vi "target_exists.vi"(8 "error in":errorcluster, 10 "Target Name":string, 11 "vsd reference":refnum<k24>) -> (0 "error out":errorcluster, 1 "target if exists":refnum<k24>, 2 "Target Exists":bool, 3 "vsd reference out":refnum<k24>)   [LabVIEW 2020]
uses:
  NationalInstruments.VeriStand.SystemDefinitionAPI
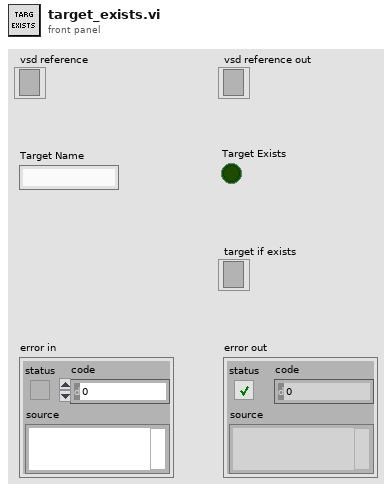
[diagram p1: front panel]
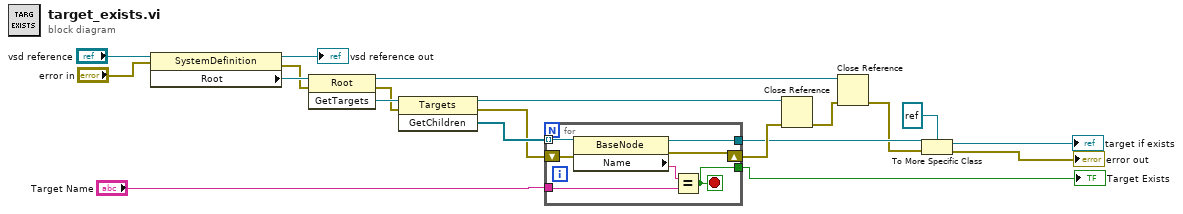
[diagram p0: block diagram]
diagram:
  n1 = property class="SystemDefinition"(reference="vsd reference", error in="error in") -> (reference out=→"vsd reference out":refnum<k24>, error out=w18:errorcluster, "Root"=w20:refnum<k24>)
  n2 = invoke class="Root" method="GetTargets"(reference=w20, error in=w18) -> (reference out=w12:refnum<k24>, error out=w6:errorcluster, "GetTargets"=w15:refnum<k24>)  [unwired: 1 in]
  n3 = invoke class="Targets" method="GetChildren"(reference=w15, error in=w6) -> (reference out=w11:refnum<k24>, error out=w13:errorcluster, "GetChildren"=w14:refnum<k24>[])  [unwired: 1 in]
  n4 = for {
    tunnel: w14 -> [w27] mode=indexing
    shift-right: [w25] -> w10
    shift-left: w13 -> [w26]
    tunnel: "Target Name" -> [w23]
    tunnel: [w22] -> w5
    tunnel: [w21] -> w7
    stop <- w21 stop-if-true
    n5 = property class="BaseNode"(reference=w27, error in=w26) -> (reference out=w22:refnum<k24>, error out=w25:errorcluster, "Name"=w24:string)
    n6 = Equal?(x=w24, y=w23) -> (x = y?=w21:bool)
  }
  "Target Exists" <- w7
  n7 = Close Reference(reference=w11, error in (no error)=w10) -> (error out=w9:errorcluster)
  n8 = Close Reference(reference=w12, error in (no error)=w9) -> (error out=w3:errorcluster)
  n9 = To More Specific Class(target class=refnum<k24> refnum, reference=w5, error in=w3) -> (specific class reference=→"target if exists":refnum<k24>, error out=→"error out":errorcluster)
